vi "dfd_Get Filter Coef Components.vi"(8 "error in (no error)":errorcluster, 11 "filter coef":T2) -> (0 "error out":errorcluster, 1 "gain":dbl, 2 "coef a (k)":dbl[](array[numeric]), 3 "coef b (v)":dbl[](array[numeric]), 5 "type":T1)   [LabVIEW 2017, in "NI_DigFilterLicensed.lvlib"]
uses:
  <vilib>/addons/Digital Filter Design/NI_DigFilterLicensed.lvlib
  <vilib>/addons/Digital Filter Design/_Objects.llb/DFD Filter Coef.ctl
  <vilib>/addons/Digital Filter Design/_Objects.llb/DFD Filter Structure Type Selector.ctl
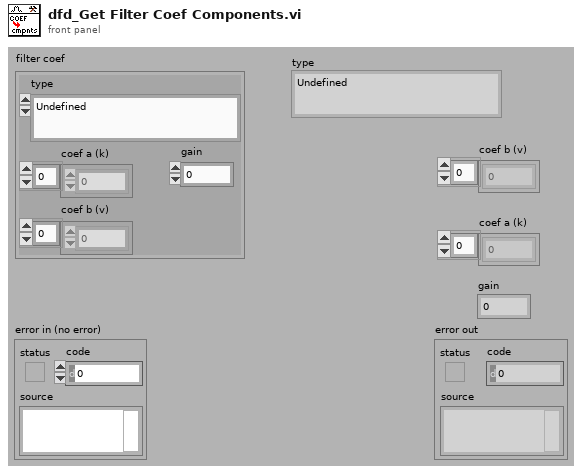
[diagram p1: front panel]
types:
  T1 = typedef "NI_DigFilterLicensed.lvlib/DFD Filter Structure Type Selector.ctl" = enum16{"Undefined", "FIR Direct Form", "FIR Direct Form Transposed", "FIR Symmetric", "FIR Antisymmetric", "IIR Direct Form I", "IIR Direct Form I Transposed", "IIR Direct Form II", "IIR Direct Form II Transposed", "IIR Cascaded Second Order Sections Form I", "IIR Cascaded Second Order Sections Form I Transposed", "IIR Cascaded Second Order Sections Form II", "IIR Cascaded Second Order Sections Form II Transposed", "Lattice Allpass (basic sections)", "Lattice Allpass (one multiplier sections)", "Lattice Allpass (normalized sections)", "Lattice AR (basic sections)", "Lattice AR (one multiplier sections)", "Lattice AR (normalized sections)", "Lattice MA (minimum phase)", "Lattice MA (maximum phase)", "Lattice ARMA (basic sections)", "Lattice ARMA (one multiplier sections)", "Lattice ARMA (normalized sections)"}
  T2 = typedef "NI_DigFilterLicensed.lvlib/DFD Filter Coef.ctl" = cluster{"type":T1, "gain":dbl, "coef a (k)":dbl[], "coef b (v)":dbl[]}
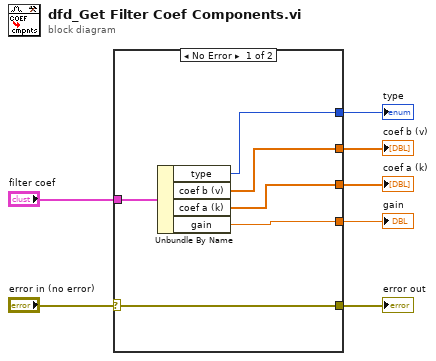
[diagram p0: block diagram]
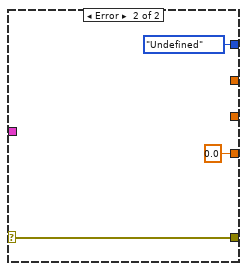
[diagram p2: hidden frame]
diagram:
  n1 = case shown="No Error" "error in (no error)" {
    selector: "error in (no error)" -> [w13 w16]
    tunnel: [w13 w16] -> w6
    tunnel: "filter coef" -> [w12 _]
    tunnel: [w11 0.0 ("gain")] -> w4
    tunnel: [w10 _] -> w3
    tunnel: [w9 _] -> w2
    tunnel: [w8 DFD_Filter_Structure_Type_Selector."Undefined" ("type")] -> w1
    frame No Error {
      n2 = Unbundle By Name(w12) -> ("type"=w8:T1, "coef b (v)"=w9:dbl[], "coef a (k)"=w10:dbl[], "gain"=w11:dbl)
    }
    frame Error {
    }
  }
  "coef a (k)" <- w3
  "coef b (v)" <- w2
  "gain" <- w4
  "type" <- w1
  "error out" <- w6
